vi "Destroy.vi"(11 "Hello World Queue in":refnum<class "Hello World Queue.lvclass">) -> (3 "Hello World Queue out":refnum<class "Hello World Queue.lvclass">)   [LabVIEW 2021, in "Hello World Queue.lvlib" / "Hello World Queue.lvclass"]
uses:
  Hello World Queue.lvclass
  Hello World Queue.lvclass/Hello World Queue.ctl
  Actor/Queue Actor/Queue Actor.lvclass
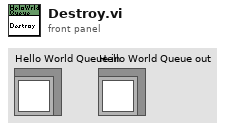
[diagram p1: front panel]
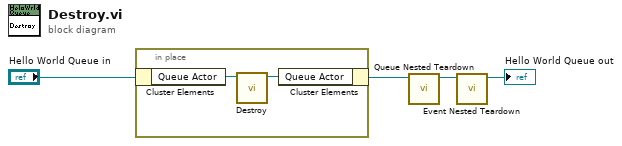
[diagram p0: block diagram]
diagram:
  n1 = in-place {
    n2 = in-place-cluster #1("Hello World Queue in") -> ("Queue Actor"=w5:refnum<class "Queue Actor.lvclass">)
    n3 = call-dynamic "Destroy.vi"("Actor in"=w5) -> ("Actor out"=w6:refnum<class "Queue Actor.lvclass">)  [unwired: 10 in]
    n4 = in-place-cluster #1("Queue Actor"=w6) -> (w2:refnum<class "Hello World Queue.lvclass">)
  }
  n5 = call-dynamic "Queue Nested Teardown.vi"("Hello World Queue in"=w2) -> ("Hello World Queue out"=w3:refnum<class "Hello World Queue.lvclass">)  [unwired: 10 in]
  n6 = call-dynamic "Event Nested Teardown.vi"("Hello World Queue in"=w3) -> ("Hello World Queue out"=→"Hello World Queue out":refnum<class "Hello World Queue.lvclass">)  [unwired: 10 in]
